vi "CVT2NamedWriteTest.vi"() -> (3 "Unit Test Framework Results":T1)   [LabVIEW 2013, in "UnitTests.lvlib"]
uses:
  UnitTests.lvlib
  <vilib>/utf/common/utf_test_result_troll.ctl
  <vilib>/utf/common/utf_test_result.ctl
  <vilib>/utf/common/utf_test_result_failure.ctl
  <vilib>/utf/common/utf_test_comparison_operators.ctl
  <vilib>/utf/common/utf_vi_tag.ctl
  <vilib>/NI/Current Value Table/DataTypes/I32_Write.vi
  <vilib>/NI/Current Value Table/DataTypes/I32_Read.vi
  <vilib>/NI/Current Value Table/Type to Enum.vi
  <vilib>/NI/Current Value Table/DataTypes/I32_Type To Enum.vi
  <vilib>/NI/Current Value Table/FGVs/CVT Globals.vi
  <vilib>/NI/Current Value Table/FGVs/Tag Memory.vi
  <vilib>/NI/Current Value Table/Memory Block.vi
  <vilib>/NI/Current Value Table/DataTypes/I32_Memory Block.vi
  <vilib>/utf/NI_UnitTestFramework.lvlib
  <vilib>/NI/Current Value Table/Current Value Table.lvlib
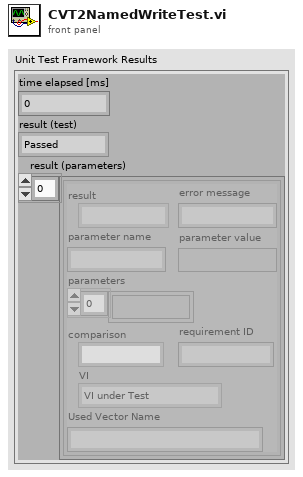
[diagram p1: front panel]
types:
  T1 = typedef "NI_UnitTestFramework.lvlib/utf_test_result_troll.ctl" = cluster{"time elapsed [ms]":u32, "result (test)":T2, "result (parameters)":T3[]}
  T2 = typedef "NI_UnitTestFramework.lvlib/utf_test_result.ctl" = enum16{"Passed", "Failed", "Error", "Skipped", "Not Processed"}
  T3 = typedef "NI_UnitTestFramework.lvlib/utf_test_result_failure.ctl" = cluster{"result":T2, "error message":string, "parameter name":string, "parameter value":variant, "parameters":variant[], "comparison":T4, "requirement ID":string, "VI":T5, "Used Vector Name":string}
  T4 = typedef "NI_UnitTestFramework.lvlib/utf_test_comparison_operators.ctl" = enum16{"=", "!=", ">", ">=", "<", "<=", "range", "symmetric tolerance", "asymmetric tolerance", "string contains", "string not contain", "array size", "string length", "array range", "by element", "array range (limit array)", "user-defined", "array contains", "array not contain", "vector length", "= (elm)", "!= (elm)", "= (case insensitive)", "!= (case insensitive)"}
  T5 = typedef "NI_UnitTestFramework.lvlib/utf_vi_tag.ctl" = enum16{"Setup VI", "VI under Test", "Teardown VI"}
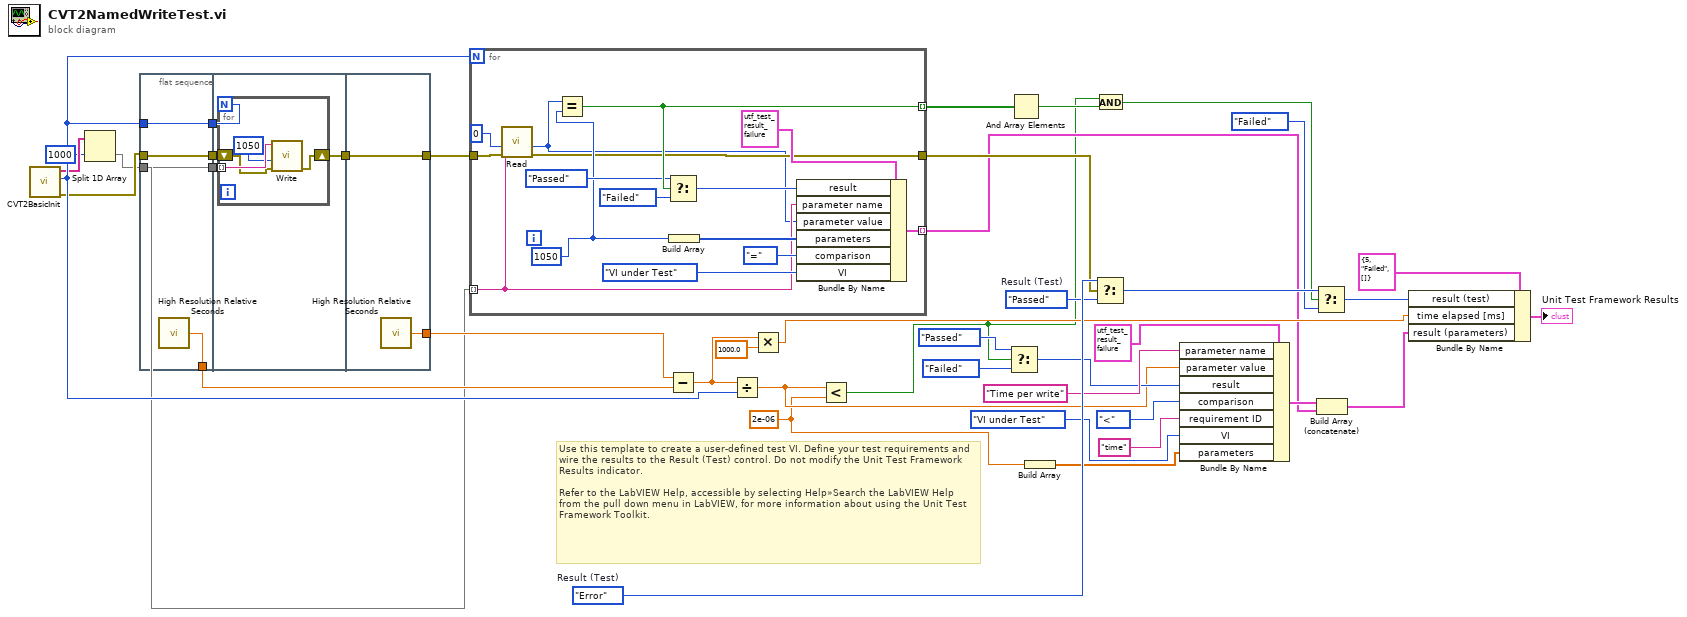
[diagram p0: block diagram]
diagram:
  w10 = 2e-06 ("y")
  w36 = utf_test_result."Error"  # Result (Test)
  w35 = utf_test_result."Passed"  # Result (Test)
  # "Use this template to create a user-defined test VI. Define your test requirements and wire the results to the Result (Test) control. Do not modify the Unit Test Framework Results indicator. \n\nRefer to the LabVIEW Help, accessible by selecting Help»Search the LabVIEW Help from the pull down menu in LabVIEW, for more information about using the Unit Test Framework Toolkit."
  n1 = call "CVT2BasicInit.vi"() -> ("error out"=w4:errorcluster, "Tags per type out"=w5:i32, "names"=w3:string[])  [unwired: 9 in]
  n2 = Split 1D Array(array=w3, index=1000) -> (second subarray=w1:string[])  [unwired: 1 out]
  n3 = flat-sequence {
    tunnel: [w45] -> w38
    tunnel: w4 -> [w42]
    tunnel: [w44] -> w30
    tunnel: w5 -> [w44]
    tunnel: w1 -> [w43]
    tunnel: [w43] -> w29
    tunnel: [w42] -> w28
    tunnel: w30 -> [w49]
    tunnel: w29 -> [w48]
    tunnel: w28 -> [w47]
    tunnel: [w46] -> w27
    tunnel: [w55] -> w39
    tunnel: w27 -> [w54]
    tunnel: [w54] -> w24
    frame #0 {
      n4 = call <vilib>:"High Resolution Relative Seconds.vi"() -> ("relative seconds"=w45:dbl)
    }
    frame #1 {
      n5 = for {
        N: w49 -> [_]
        tunnel: w48 -> [w53] mode=indexing
        shift-right: [w50] -> w46
        shift-left: w47 -> [w52]
        n6 = call-poly <vilib>:"Write.vi"("error in (no error)"=w52, "Value"=1050, "Tag Name"=w53) -> ("error out"=w50:errorcluster)  [unwired: 8 in]
      }
    }
    frame #2 {
      n7 = call <vilib>:"High Resolution Relative Seconds.vi"() -> ("relative seconds"=w55:dbl)
    }
  }
  n8 = for {
    N: w5 -> [_]
    tunnel: w1 -> [w59] mode=indexing
    tunnel: w24 -> [w60]
    tunnel: [w58] -> w23
    tunnel: [w68] -> w22 mode=indexing
    tunnel: [w64] -> w8 mode=indexing
    w61 = 1050 ("Value")
    n9 = call-poly <vilib>:"Read.vi"("error in (no error)"=w60, "Default"=0, "Tag Name"=w59) -> ("error out"=w58:errorcluster, "Value"=w57:i32)  [unwired: 7 in]
    n10 = Equal?(x=w57, y=w61) -> (x = y?=w68:bool)
    n11 = Select(t=utf_test_result."Passed" ("result"), s=w68, f=utf_test_result."Failed" ("result")) -> (s? t:f=w65:T2)
    n12 = Build Array(w61) -> (w62:i32[])
    n13 = Bundle By Name(cluster=T3 {"result"=enum."Passed", "error message"="", "parameter name"="", "parameter value"=variant, "parameters"=[], "comparison"=enum."=", "requirement ID"="", "VI"=enum."Setup VI", "Used Vector Name"=""} ("Unit Test Framework - result (parameters)"), "result"=w65, "parameter name"=w59, "parameter value"=w57, "parameters"=w62, "comparison"=utf_test_comparison_operators."=", "VI"=utf_vi_tag."VI under Test") -> (w64:T3)
  }
  n14 = Subtract(x=w39, y=w38) -> (x-y=w26:dbl)
  n15 = Divide(x=w26, y=w5) -> (x/y=w13:dbl)
  n16 = Multiply(x=w26, y=1000.0) -> (x*y=w31:dbl)
  n17 = Less?(x=w13, y=w10) -> (x < y?=w6:bool)
  n18 = Select(t=utf_test_result."Passed" ("result"), s=w6, f=utf_test_result."Failed" ("result")) -> (s? t:f=w14:T2)
  n19 = And Array Elements(Boolean array=w22) -> (logical AND=w21:bool)
  n20 = Build Array(w10) -> (w9:dbl[])
  n21 = Select(t=w36, s=w23, f=w35) -> (s? t:f=w20:T2)
  n22 = And(x=w6, y=w21) -> (x .and. y?=w7:bool)
  n23 = Bundle By Name(cluster=T3 {"result"=enum."Passed", "error message"="", "parameter name"="", "parameter value"=variant, "parameters"=[], "comparison"=enum."=", "requirement ID"="", "VI"=enum."Setup VI", "Used Vector Name"=""} ("Unit Test Framework - result (parameters)"), "parameter name"="Time per write", "parameter value"=w13, "result"=w14, "comparison"=utf_test_comparison_operators."<", "requirement ID"="time", "VI"=utf_vi_tag."VI under Test", "parameters"=w9) -> (w34:T3)
  n24 = Select(t=w20, s=w7, f=utf_test_result."Failed") -> (s? t:f=w18:T2)
  n25 = Build Array (concatenate)(w34, w8) -> (w33:T3[])
  n26 = Bundle By Name(cluster=T1 {"time elapsed [ms]"=5, "result (test)"=enum."Failed", "result (parameters)"=[]} ("Unit Test Framework - Result"), "result (test)"=w18, "time elapsed [ms]"=w31, "result (parameters)"=w33) -> (→"Unit Test Framework Results":T1)
